vi "SpectrumAnalyzer.vi"() -> ()   [LabVIEW 2024]
uses:
  <instrlib>/Rohde&Schwarz Spectrum Analyzer/Rohde&Schwarz Spectrum Analyzer.lvlib
  <vilib>/Utility/xml.llb/Write to XML File(string).vi
  <instrlib>/_Template - Spectrum Analyzer/Template - Spectrum Analyzer.lvlib
  <vilib>/Utility/xml.llb/Write to XML File(array).vi
panel:
  in  "EVM (dB)":i32(ring)=8 items=["dB"=8, "%"=13]
  out "Trace Waveform":T1(graph)
  out "VISA resource name out":refnum<visa-resource-name>
  in  "format string 3":string
  in  "format string 2":string
  in  "format string":string
  in  "OPEN":path
  in  "Ref Level Offset":dbl
  in  "Attenuation":dbl
  in  "Centre freq":dbl caption="Centre Freq"
  in  "Ref Level":dbl
  in  "Input Imp":dbl
  in  "Stop Freq":dbl
  in  "Start Freq":dbl
  in  "Sweep Time":dbl caption="Time Sweep"
  out "error out":errorcluster {"code" format="%.0x"}
  in  "Video bandwith":dbl caption="Video BW"
  in  "Resolution bandwith":dbl caption="Resolution BW"
  out "PSD":dbl format="%^.3e"
  out "Frequency":dbl caption="Frequency (Peak Search)" format="%^.3e"
  in  "error in (no error)":errorcluster {"code" format="%.0x"}
  in  "VISA resource name":refnum<visa-resource-name>="GPIB::20"
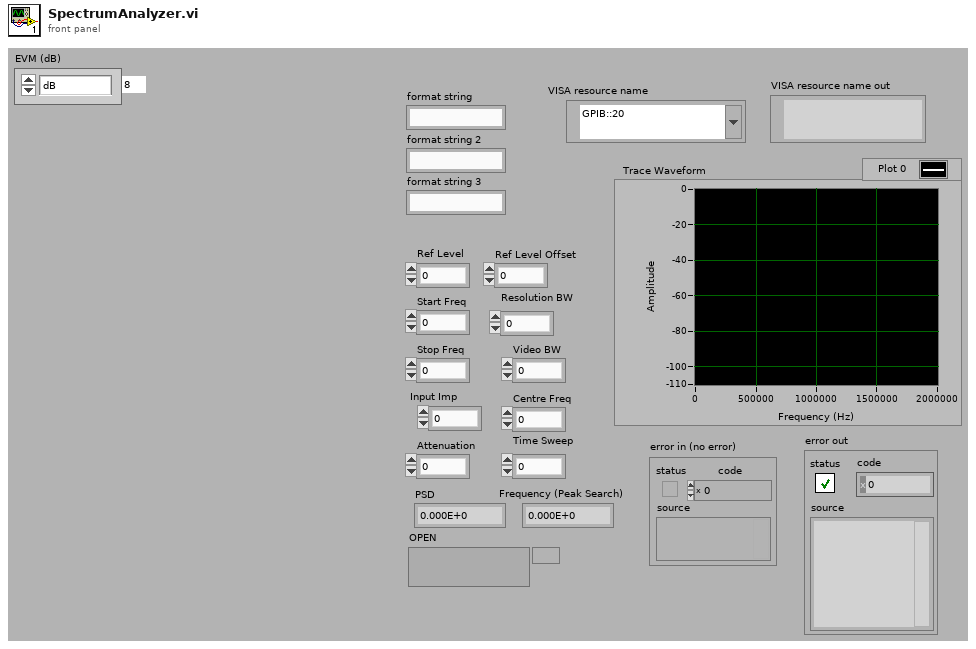
[diagram p1: front panel]
types:
  T1 = cluster{"Start Frequency (0 Hz)":dbl, dbl, "Trace":sgl[]}
  T2 = cluster{"Initial X":dbl, "X Increment":dbl, "Trace Array":sgl[]}
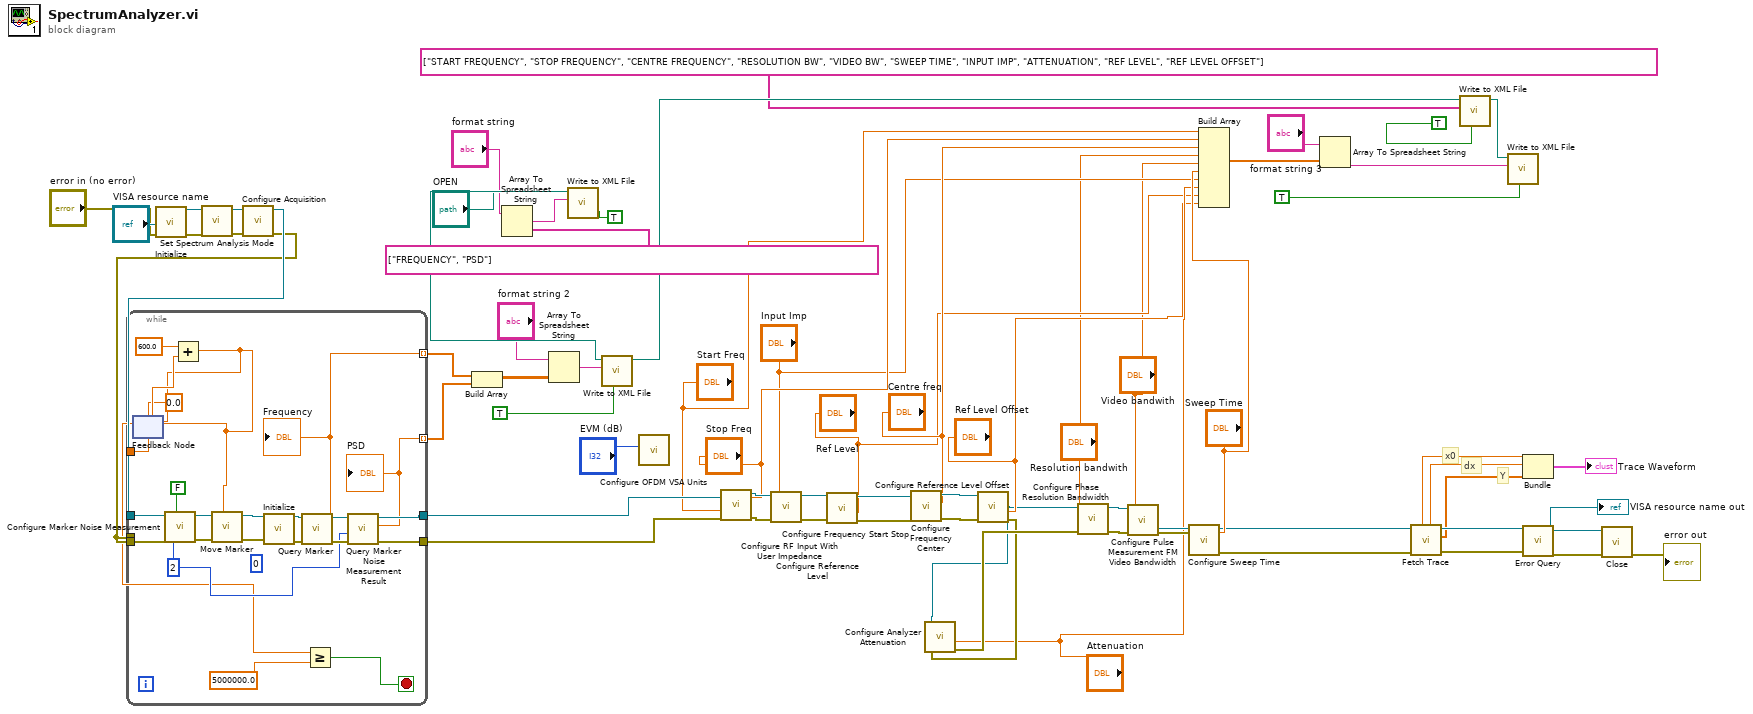
[diagram p0: block diagram]
diagram:
  # "Y"
  # "dx"
  # "x0"
  n1 = call <instrlib>:"Initialize.vi"("VISA resource name"="VISA resource name", "error in (no error)"="error in (no error)") -> ("VISA resource name out"=w64:refnum<visa-resource-name>, "error out"=w65:errorcluster)  [unwired: 12 in]
  n2 = call <instrlib>:"Set Spectrum Analysis Mode.vi"("error in (no error)"=w65, "VISA resource name"=w64) -> ("error out"=w62:errorcluster, "VISA resource name out"=w63:refnum<visa-resource-name>)  [unwired: 8 in]
  n3 = call <instrlib>:"Configure Acquisition.vi"("error in (no error)"=w62, "VISA resource name"=w63) -> ("error out"=w23:errorcluster, "VISA resource name out"=w61:refnum<visa-resource-name>)  [unwired: 8 in]
  n4 = while {
    tunnel: w23 -> [_]
    tunnel: w61 -> [w73]
    tunnel: [w80] -> w17
    tunnel: [w79] -> w16
    tunnel: [w71] -> w45 mode=indexing
    tunnel: [w68] -> w46 mode=indexing
    tunnel: w23 -> [w85]
    tunnel: [w74] -> _
    stop <- w89 stop-if-true
    (unwired) 0 ("Timeout (15000)")
    w74 = 0.0
    w70 = 2 ("Marker (1)")
    n5 = feedback #1(w74) -> (w86:dbl)
    n6 = call <instrlib>:"Configure Marker Noise Measurement.vi"("State (F: Off)"=FALSE ("State (Off)"), "error in (no error)"=w85, "Marker (1)"=w70, "VISA resource name"=w73) -> ("error out"=w83:errorcluster, "VISA resource name out"=w84:refnum<visa-resource-name>)  [unwired: 6 in]
    n7 = Add(x=600.0, y=w86) -> (x+y=w69:dbl)
    n8 = feedback-in #1(w69) -> ()
    n9 = call <instrlib>:"Move Marker.vi"("Marker Position (0.0)"=w69, "error in (no error)"=w83, "VISA resource name"=w84) -> ("error out"=w81:errorcluster, "VISA resource name out"=w82:refnum<visa-resource-name>)  [unwired: 7 in]
    n10 = call <instrlib>:"Initialize.vi"("VISA resource name"=w82, "error in (no error)"=w81) -> ("VISA resource name out"=w77:refnum<visa-resource-name>, "error out"=w78:errorcluster)  [unwired: 12 in]
    n11 = call <instrlib>:"Query Marker.vi"("error in (no error)"=w78, "VISA resource name"=w77) -> ("error out"=w75:errorcluster, "Marker Position"=w68:dbl, "VISA resource name out"=w76:refnum<visa-resource-name>)  [unwired: 6 in, 1 out]
    "Frequency" <- w68
    n12 = Greater Or Equal?(x=w69, y=5000000.0) -> (x >= y?=w89:bool)
    n13 = call <instrlib>:"Query Marker Noise Measurement Result.vi"("error in (no error)"=w75, "Marker (1)"=w70, "VISA resource name"=w76) -> ("error out"=w79:errorcluster, "Result"=w71:dbl, "VISA resource name out"=w80:refnum<visa-resource-name>)  [unwired: 6 in]
    "PSD" <- w71
  }
  n14 = Build Array(w46, w45) -> (w24:dbl[][])
  n15 = Array To Spreadsheet String(array=string[] ["FREQUENCY", "PSD"] ("1D data"), 3:"format string") -> (spreadsheet string=w26:string)  [unwired: 1 in]
  n16 = Array To Spreadsheet String(array=w24, 3:"format string 2") -> (spreadsheet string=w25:string)  [unwired: 1 in]
  n17 = call-poly <vilib>:"Write to XML File.vi"("Standalone? (T)"=TRUE, "XML Input"=w26, "XML File Path"="OPEN") -> ("XML File Path(duplicate)"=w44:path)  [unwired: 6 in, 2 out]
  n18 = call-poly <vilib>:"Write to XML File.vi"("Standalone? (T)"=TRUE ("append to file? (new file:F)"), "XML Input"=w25, "XML File Path"=w44) -> ("XML File Path(duplicate)"=w34:path)  [unwired: 6 in, 2 out]
  n19 = call <instrlib>:"Configure OFDM VSA Units.vi"("EVM (dB)"="EVM (dB)") -> ()  [unwired: 9 in, 2 out]
  n20 = call <instrlib>:"Configure Frequency Start Stop.vi"("Stop Frequency (0Hz)"="Stop Freq", "error in (no error)"=w16, "Start Frequency (0Hz)"="Start Freq", "VISA resource name"=w17) -> ("error out"=w55:errorcluster, "VISA resource name out"=w56:refnum<visa-resource-name>)  [unwired: 6 in]
  n21 = call <instrlib>:"Configure RF Input With User Impedance.vi"("error in (no error)"=w55, "Impedance (50.0)"="Input Imp", "VISA resource name"=w56) -> ("error out"=w53:errorcluster, "VISA resource name out"=w54:refnum<visa-resource-name>)  [unwired: 7 in]
  n22 = call <instrlib>:"Configure Reference Level.vi"("error in (no error)"=w53, "Reference Level (-20.0)"="Ref Level", "VISA resource name"=w54) -> ("error out"=w51:errorcluster, "VISA resource name out"=w52:refnum<visa-resource-name>)  [unwired: 7 in]
  n23 = call <instrlib>:"Configure Frequency Center.vi"("error in (no error)"=w51, "Center Frequency (0Hz)"="Centre freq", "VISA resource name"=w52) -> ("error out"=w48:errorcluster, "VISA resource name out"=w49:refnum<visa-resource-name>)  [unwired: 7 in]
  n24 = call <instrlib>:"Configure Reference Level Offset.vi"("error in (no error)"=w48, "Reference Level Offset (0.0)"="Ref Level Offset", "VISA resource name"=w49) -> ("error out"=w47:errorcluster, "VISA resource name out"=w14:refnum<visa-resource-name>)  [unwired: 7 in]
  n25 = call <instrlib>:"Configure Analyzer Attenuation.vi"("error in (no error)"=w47, "Attenuation (10)"="Attenuation", "VISA resource name"=w14) -> ("error out"=w50:errorcluster)  [unwired: 7 in, 1 out]
  n26 = call <instrlib>:"Configure Phase Resolution Bandwidth.vi"("error in (no error)"=w50, "RBW (10.0)"="Resolution bandwith", "VISA resource name"=w14) -> ("error out"=w60:errorcluster, "VISA resource name out"=w57:refnum<visa-resource-name>)  [unwired: 7 in]
  n27 = call <instrlib>:"Configure Pulse Measurement FM Video Bandwidth.vi"("error in (no error)"=w60, "FM Video Bandwidth (None)"="Video bandwith", "VISA resource name"=w57) -> ("error out"=w58:errorcluster, "VISA resource name out"=w59:refnum<visa-resource-name>)  [unwired: 7 in]
  n28 = call <instrlib>:"Configure Sweep Time.vi"("Sweep Time (0.268)"="Sweep Time", "error in (no error)"=w58, "VISA resource name"=w59) -> ("error out"=w7:errorcluster, "VISA resource name out"=w6:refnum<visa-resource-name>)  [unwired: 7 in]
  n29 = Build Array("Start Freq", "Stop Freq", "Centre freq", "Resolution bandwith", "Video bandwith", "Sweep Time", "Input Imp", "Attenuation", "Ref Level", "Ref Level Offset") -> (w28:dbl[])
  n30 = Array To Spreadsheet String(array=w28, 3:"format string 3") -> (spreadsheet string=w29:string)  [unwired: 1 in]
  n31 = call <instrlib>:"Fetch Trace.vi"("error in (no error)"=w7, "VISA resource name"=w6) -> ("error out"=w12:errorcluster, "Trace Array"=w8:sgl[], "VISA resource name out"=w13:refnum<visa-resource-name>, "X Increment"=w11:dbl, "Initial X"=w10:dbl)  [unwired: 5 in]
  n32 = call-poly <vilib>:"Write to XML File.vi"("Standalone? (T)"=TRUE ("append to file? (new file:F)"), "XML Input"=string[] ["START FREQUENCY", "STOP FREQUENCY", "CENTRE FREQUENCY", "RESOLUTION BW", "VIDEO BW", "SWEEP TIME", "INPUT IMP", "ATTENUATION", "REF LEVEL", "REF LEVEL OFFSET"] ("1D data"), "XML File Path"=w34) -> ("XML File Path"=w35:path)  [unwired: 6 in, 2 out]
  n33 = call-poly <vilib>:"Write to XML File.vi"("Standalone? (T)"=TRUE ("append to file? (new file:F)"), "XML Input"=w29, "XML File Path"=w35) -> ()  [unwired: 6 in, 3 out]
  n34 = Bundle("Initial X"=w10, "X Increment"=w11, "Trace Array"=w8) -> (→"Trace Waveform":T2)  [unwired: 1 in]
  n35 = call <instrlib>:"Error Query.vi"("error in (no error)"=w12, "VISA resource name"=w13) -> ("error out"=w5:errorcluster, "VISA resource name out"=w3:refnum<visa-resource-name>)  [unwired: 6 in, 2 out]
  "VISA resource name out" <- w3
  n36 = call <instrlib>:"Close.vi"("error in (no error)"=w5, "VISA resource name"=w3) -> ("error out"=→"error out":errorcluster)  [unwired: 9 in]
